vi "CPP_Aeroprobe_dT-Unified-kag.vi"() -> (5 "Plug in titles":string[](array[string]), 7 "Plug in values":string[](array[string]))   [LabVIEW 2016]
uses:
  ADAM Client/Sub VIs/ADAM Controls/Ch_description_ADAM.ctl
  ADAM Client/Sub VIs/ADAM Controls/Module_type_ADAM.ctl
  ADAM Client/Sub VIs/ADAM Controls/Function_ADAM.ctl
  ADAM Client/Sub VIs/ADAM Controls/Channel_State.ctl
  ADAM Client/Sub VIs/ADAM Controls/Calib_type_ADAM.ctl
  ADAM Client/Sub VIs/ADAM Controls/Address.ctl
  ADAM Client/Sub VIs/ADAM Controls/Update_scan_value.ctl
  <vilib>/Analysis/baseanly.llb/Mean (DBL).vi
  Globals/Constants_global.vi
  Globals/Meas_global.vi
  Globals/Trav_pos_global.vi
  <vilib>/Utility/file.llb/Write Delimited Spreadsheet (DBL).vi
  <vilib>/Analysis/NI_AALBase.lvlib
panel:
  out "MDZeroesVars":string[](array[string])
  out "MDZeroesMeans":string[](array[string])
  out "AeroFlow Output":cluster{string, string}[](array[cluster]) caption="Plug In Titles                                   Plug In Values"
  out "ZeroMeans&Vars":dbl[](array[numeric])
  out "ADAM Chs":T1[](array[typedef]) {"Duty" format="%.0b"; "D" format="%#_5g"; "C" format="%#_5g"; "B" format="%#_5g"; "A" format="%#_5g"}
  in  "Probe Orientation":u16(ring)=90 items=["Horizontal"=0, "Diagonal"=45, "Vertical"=90]
  in  "Probe Type":u16(ring)=12 items=["5-Hole Probe"=5, "OmniProbe"=12]
  in  "SaveTimeSeries?":bool
  in  "Mode":enum32{"Measure", "Take Zeroes"}(radio)
  in  "RunManually?":bool
  in  "MeanOrFull":bool
  in  "Graphs":bool
  in  "Downsampler":i32=80
  in  "Calibration Folder Path":path
  in  "Correction File Path":path
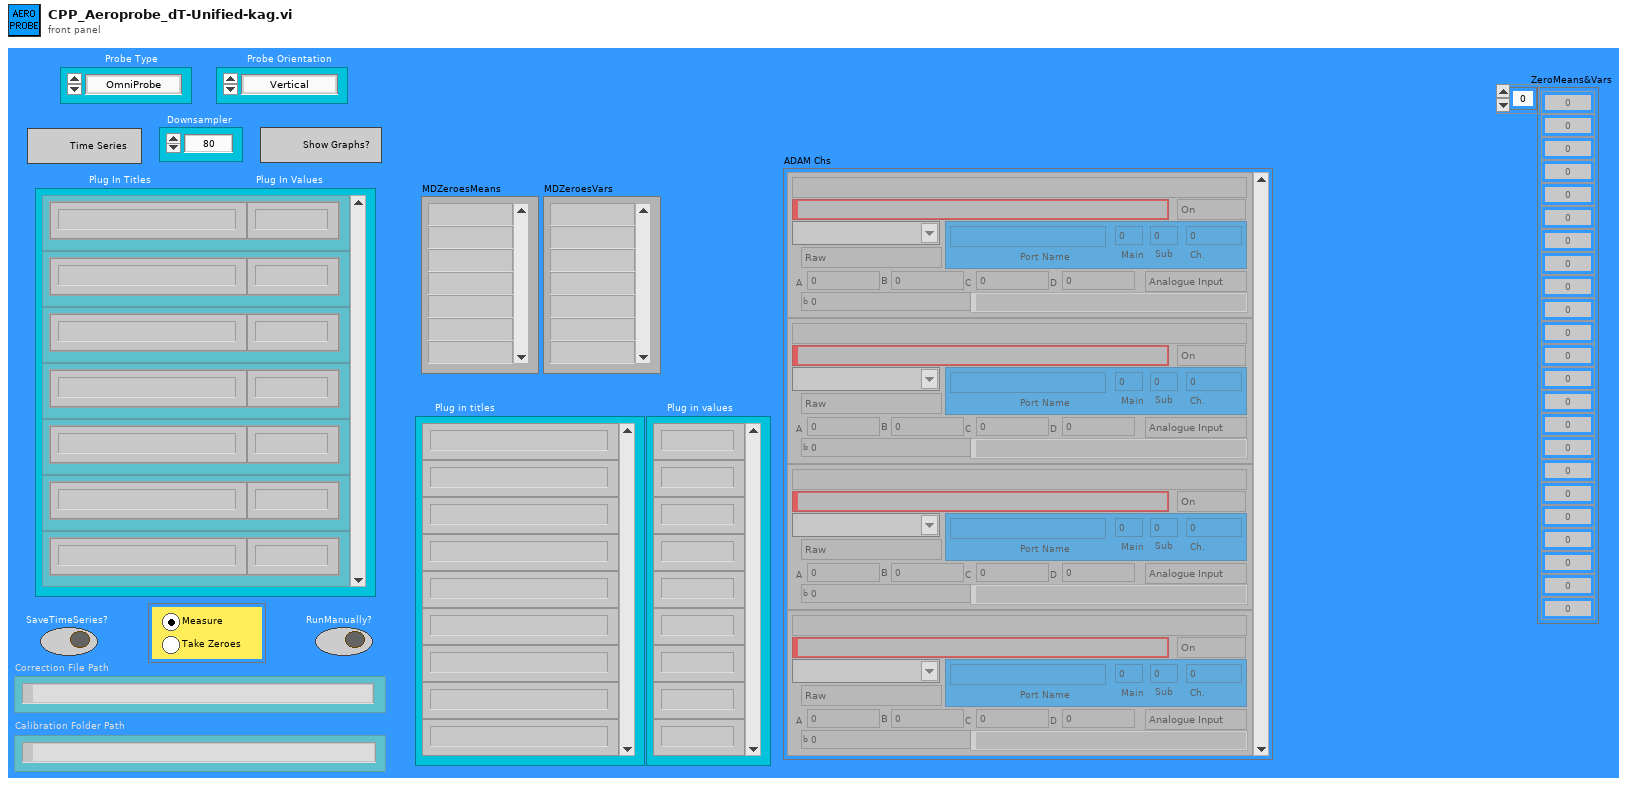
[diagram p1: front panel]
types:
  T1 = typedef "Ch_description_ADAM.ctl" = cluster{"Ch Name":string, "Type":T2, "Function":T3, "Ch State":T4, "Calibration type":T5, "A":dbl, "B":dbl, "C":dbl, "D":dbl, "Comments":string, "Address":T6, "String":string, "Duty":u16}
  T2 = typedef "Module_type_ADAM.ctl" = string
  T3 = typedef "Function_ADAM.ctl" = enum16{"Analogue Input", "Digital Input", "Event counter", "Event rate", "Analogue Output", "Digital Output", "Relay Output"}
  T4 = typedef "Channel_State.ctl" = enum16{"On", "Off", "Always On", "Always Off"}
  T5 = typedef "Calib_type_ADAM.ctl" = enum16{"Raw", "Bx + A", "Cx^2 + Bx + A", "Dx^3 + Cx^2 + Bx + A", "In Band", "Hi-Tec Q", "Hi-Tec M_dot", "Text"}
  T6 = typedef "Address.ctl" = cluster{"Main":i32, "Ch.":i32, "Sub":i32, "Port Name":string}
  T7 = enum16{"Save no data", "Save data in new files", "Save data in existing files"}
  T8 = typedef "Post_Process.ctl" = enum16{"Take New Data", "Post Process Raw Data File"}
  T9 = typedef "Analysis_info_cluster.ctl" = cluster{"Colour":u32, "Inst type":T10, "Inst name":string, "Symbol":string, "Code name":string, "Extra Info":string, "Inst Array":T11, "Extra Titles":string[], "Extra Values":string[], "U":dbl, "u^2":dbl, "u^3":dbl, "u^4":dbl, "Skew_u":dbl, "Kurt_u":dbl, "Sd Error in Mean":dbl, "% u'/U":dbl, "X":dbl, "Y":dbl, "Z":dbl, "Timescale integral to 25%":dbl, "Sd Error in Variance":dbl, "Calib File":path, "Calib Constants":dbl[], "Output Position":bool, "Full Stats":bool, "Av Sampling Rate":dbl, "Av No of Samples":dbl, "Total Meas Time (s)":dbl, "ADAM Ch Name":string, "Max value":dbl, "Min value":dbl}
  T10 = typedef "Inst_type.ctl" = enum16{"Propeller anemometer", "Raw voltage", "Pressure Transducer", "Pitot-static tube", "Preston tube", "Hot wire", "Cross wire 1", "Cross wire 2", "Generic Linear", "Generic Polynomial", "Generic BackPoly", "Fast FID", "Thermocouple", "Cold wire", "Pulsed Wire", "LDA Vel", "LDA Tran time", "LDA Arr time", "Microphone"}
  T11 = typedef "Instrument_Array.ctl" = enum16{"PWA", "LDA", "Analogue"}
  T12 = typedef "Traverse_cluster.ctl" = cluster{"Start X":sgl, "Start Y":sgl, "Start Z":sgl, "End X":sgl, "End Y":sgl, "End Z":sgl, "No. of pts.":i32, "Spacing":T13, "Filename":path, "Tunnel Speed":dbl, "Averaging time (min)":dbl, "Extra Commands":string, "Carrier_1 Q (l/min)":dbl, "Carrier_2 Q (l/min)":dbl, "Trace Gas Concentration (%)":dbl, "Specific Arguments":string, "Comments":string, "Row No":i32, "Row Type Selector":T14, "Completion time":string, "Row Duration (mins)":dbl, "No. of Valid pts.":i32, "Meas Setup File":string}
  T13 = typedef "Spacing.ctl" = enum16{"Linear", "Log", "Gauss", "Specified", "N/A"}
  T14 = typedef "Multi_run_mode.ctl" = enum16{"Move Traverse Only", "Set Tunnel Speed Only", "Set Source Only", "Set Measurement Conditions", "Single Measurement", "Vertical Profile", "Lateral Profile", "Longitudinal Profile", "Explore Volume", "Multi-Axis Profile", "Auto Calibrate", "Meas Fast FID Bkgnd", "Check Beam Power", "Scanning Valve Measurement", "Run VI Named:", "Set ADAM Ch", "Wait (minutes)", "Send Message", "Synchronize With:", "Fall Back to this Row", "Turn Off Row Repeating", "Blank Row", "Traverse 3D Volume"}
  T15 = typedef "Update_scan_value.ctl" = cluster{"Channel Name":string, "New Value":dbl}
  T16 = typedef "Time_Trace_Cluster.ctl" = cluster{"Weighting":dbl[], "Time (s)":dbl[], "Voltage":dbl[], "Eng Values":dbl[]}
  T17 = typedef "GoodArray.ctl" = bool[]
  T18 = typedef "SanityCluster.ctl" = cluster{"PressureErrors":bool[][], "Plug in titles":string[]}
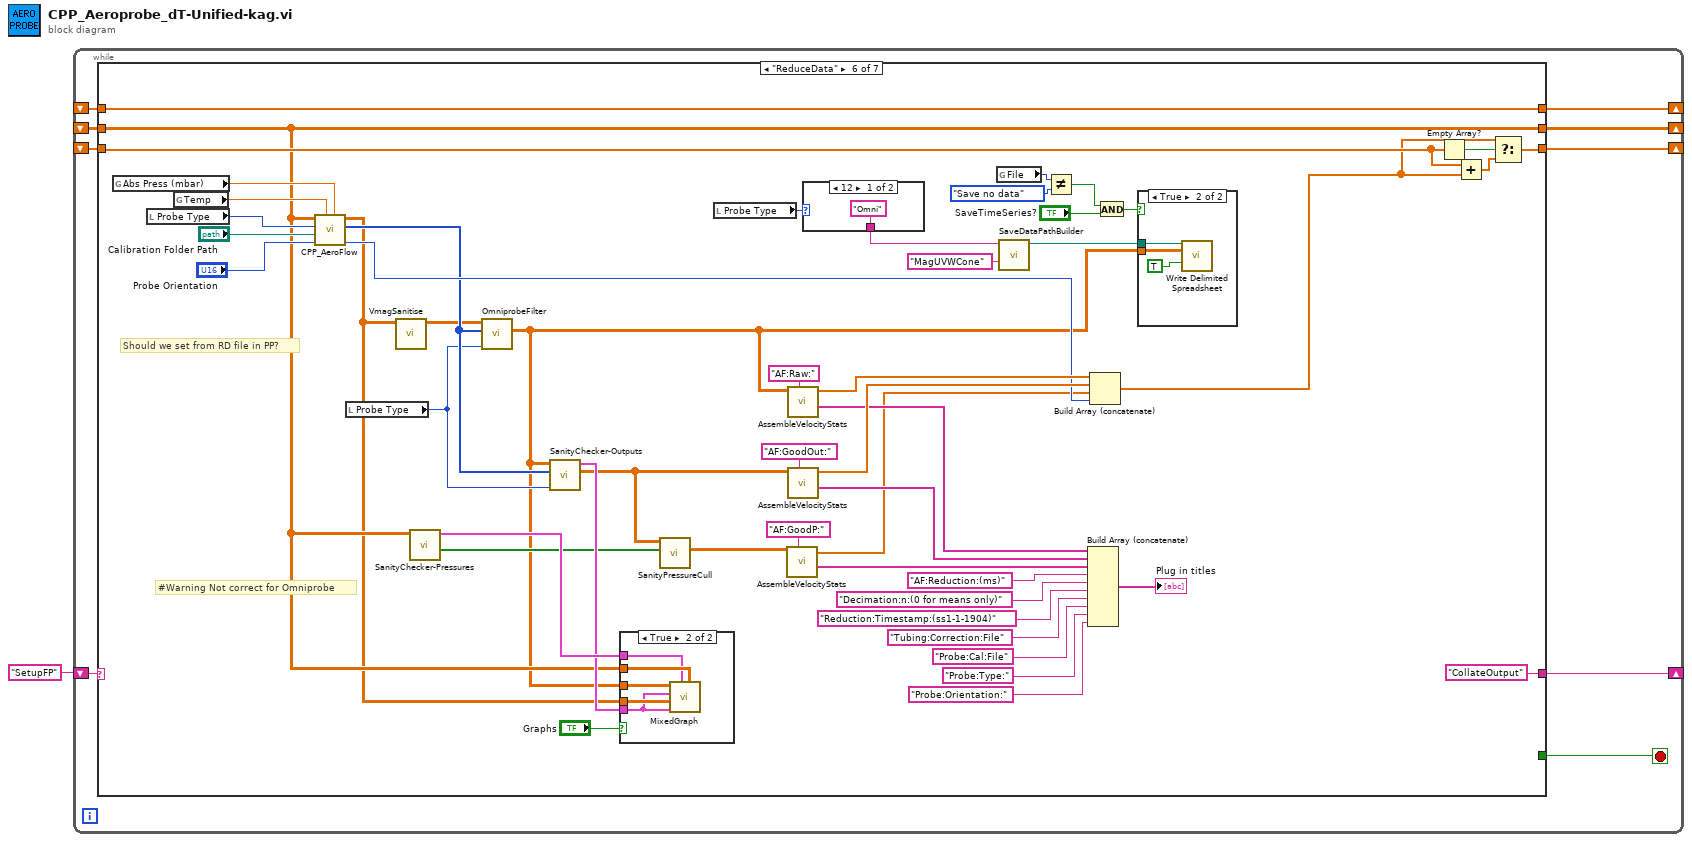
[diagram p0: block diagram]
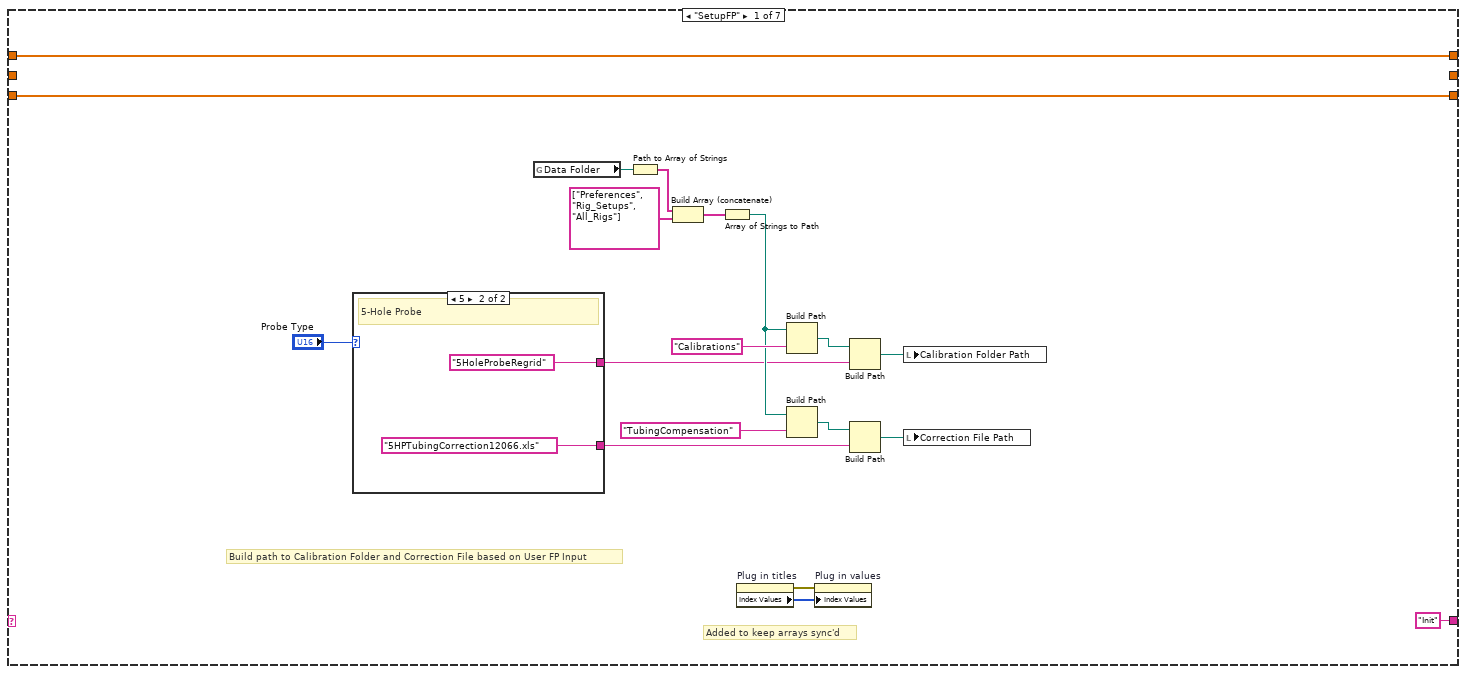
[diagram p2: hidden frame]
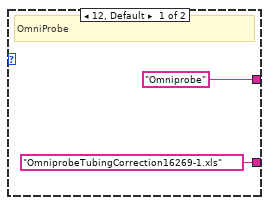
[diagram p3: hidden frame]
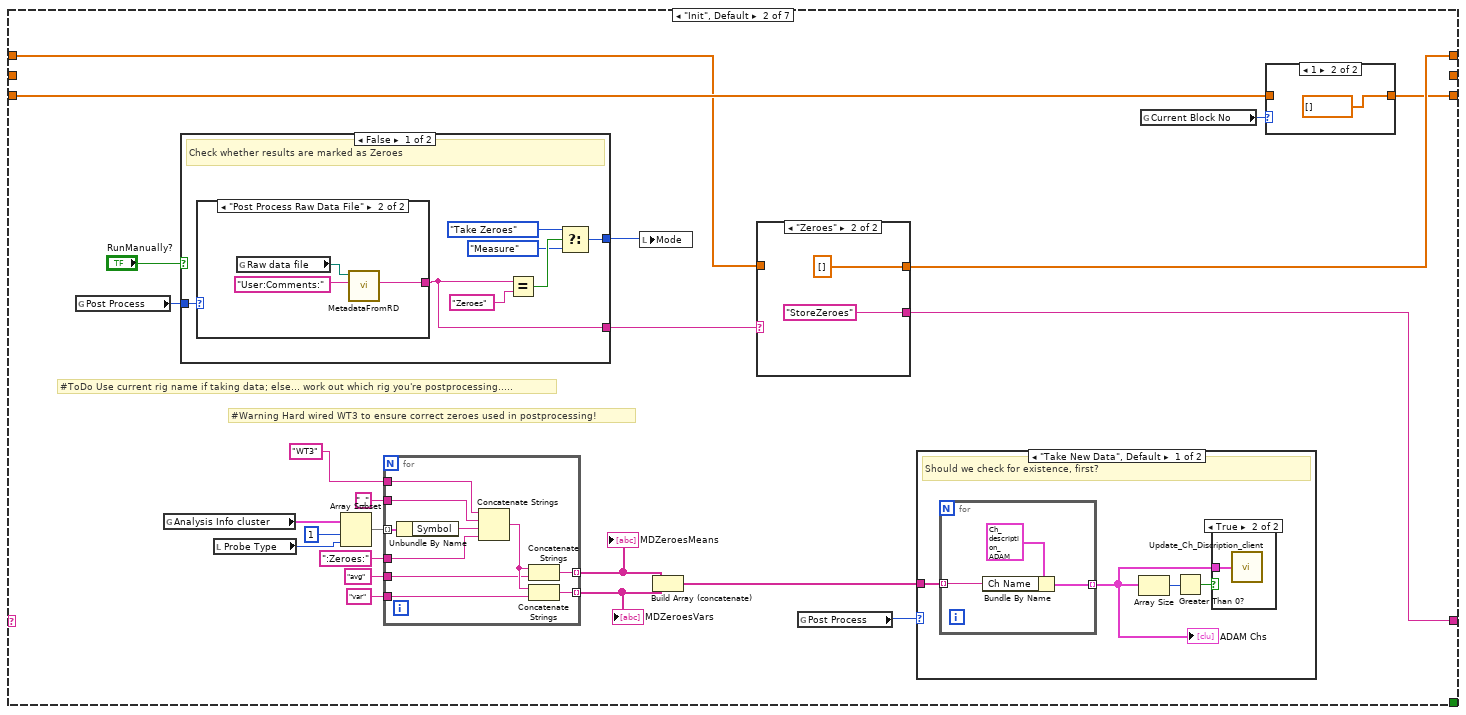
[diagram p4: hidden frame]
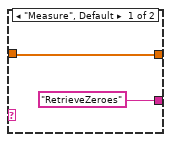
[diagram p7: hidden frame]
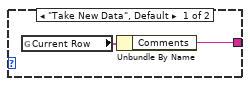
[diagram p8: hidden frame]
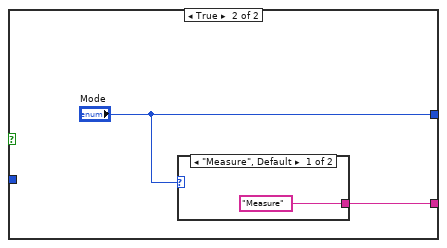
[diagram p9: hidden frame]
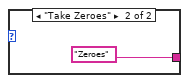
[diagram p10: hidden frame]
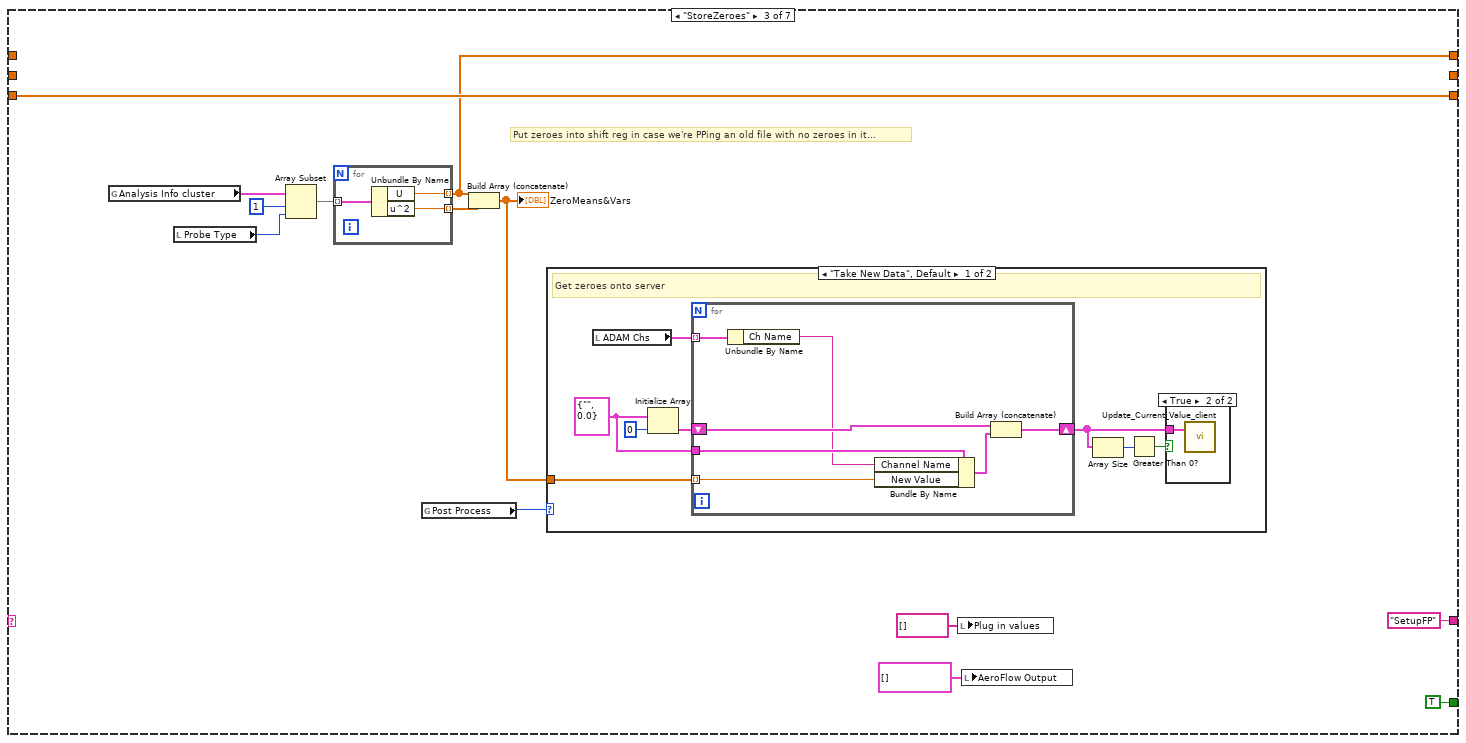
[diagram p12: hidden frame]
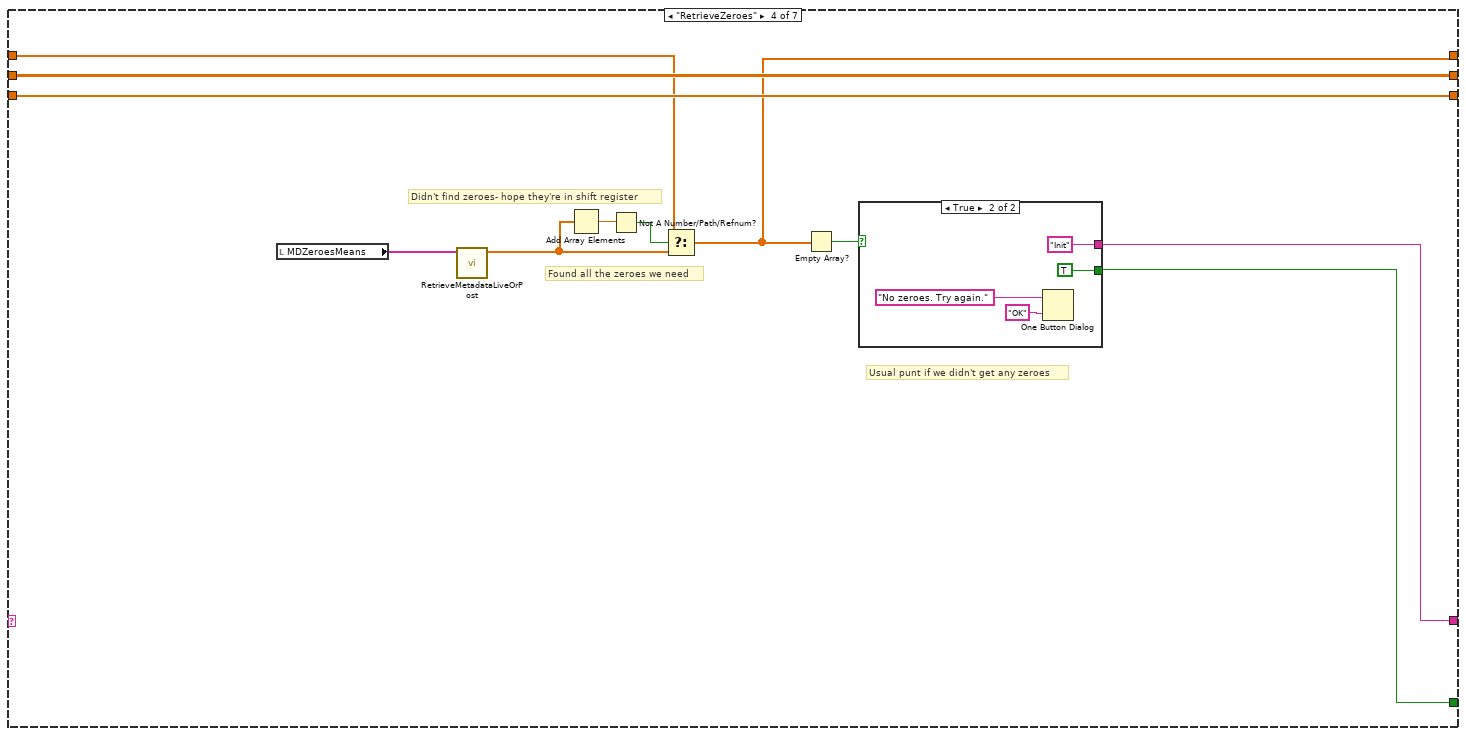
[diagram p15: hidden frame]
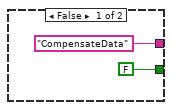
[diagram p16: hidden frame]
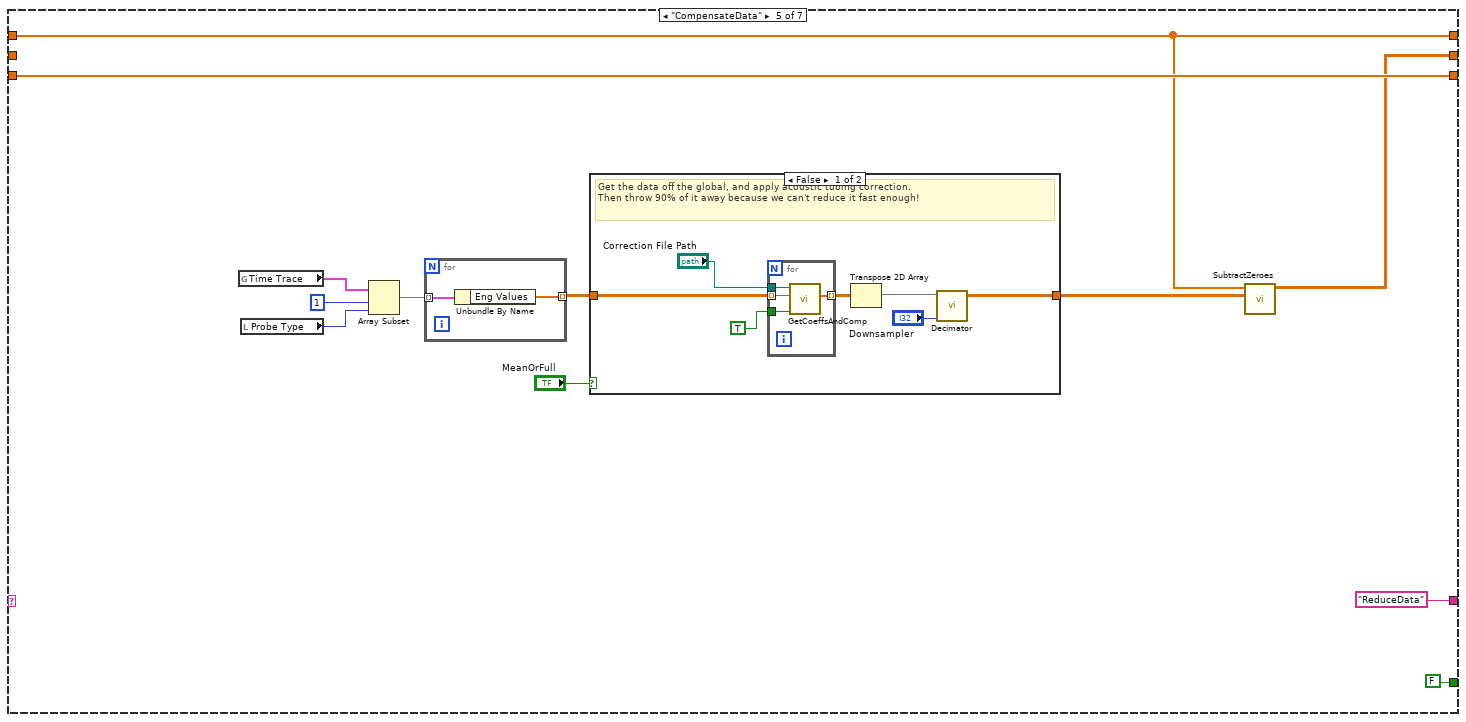
[diagram p17: hidden frame]
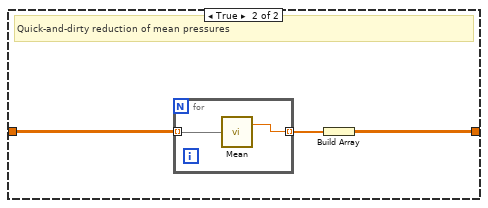
[diagram p18: hidden frame]
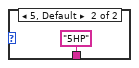
[diagram p19: hidden frame]
diagram:
  n1 = while {
    shift-right: [w9] -> _
    shift-left: "SetupFP" -> [w10]
    shift-right: [w8] -> _
    shift-left: _ -> [w7]
    shift-right: [w6] -> _
    shift-left: _ -> [w5]
    shift-right: [w3] -> _
    shift-left: _ -> [w2]
    stop <- w4 stop-if-true
    n2 = case shown="\"ReduceData\"" w10 {
      tunnel: ["Init" w39 "SetupFP" w134 "ReduceData" "CollateOutput" "Init"] -> w9
      tunnel: [w29 w56 w103 w129 w155 w225 w262] -> w8
      tunnel: w7 -> [w29 w40 _ w131 w155 w225 w262]
      tunnel: [w28 w55 w109 w139 w157 w221 w256] -> w6
      tunnel: w5 -> [w28 w54 w109 w139 w157 w224 w256]
      tunnel: [_ _ TRUE w133 FALSE _ TRUE] -> w4
      tunnel: [_ _ _ w138 w152 w181 w258] -> w3
      tunnel: w2 -> [_ _ _ w138 _ w181 w258]
      frame "SetupFP" {
        # "Added to keep arrays sync'd"
        # "Build path to Calibration Folder and Correction File based on User FP Input"
        n3 = case shown="5" "Probe Type" {
          tunnel: ["OmniprobeTubingCorrection16269-1.xls" ("Tubing Compensation File") "5HPTubingCorrection12066.xls" ("Tubing Compensation File")] -> w18
          tunnel: ["Omniprobe" ("Calibration Folder") "5HoleProbeRegrid" ("Calibration Folder")] -> w17
          frame 12, Default {
            # "OmniProbe"
          }
          frame 5 {
            # "5-Hole Probe"
          }
        }
        n4 = global read "Constants_global.vi" "Data Folder"() -> (w23:path)
        n5 = Path to Array of Strings(0:w23) -> (2:w26:string[])  [unwired: 1 out]
        n6 = Build Array (concatenate)(w26, string[] ["Preferences", "Rig_Setups", "All_Rigs"] ("array of strings 3")) -> (w24:string[])
        n7 = Array of Strings to Path(0:w24) -> (2:w20:path)  [unwired: 1 in]
        n8 = property on="Plug in titles" class="Arr (strict)"() -> (error out=w11:errorcluster, "Index Values"=w12:u32[])  [unwired: 2 in, 1 out]
        n9 = Build Path(base path=w20, name or relative path="Calibrations") -> (appended path=w15:path)
        n10 = Build Path(base path=w20, name or relative path="TubingCompensation") -> (appended path=w16:path)
        n11 = property on="Plug in values" class="Arr (strict)"(error in=w11, "Index Values"=w12) -> ()  [unwired: 1 in, 2 out]
        n12 = Build Path(base path=w15, name or relative path=w17) -> (appended path=w14:path)
        n13 = Build Path(base path=w16, name or relative path=w18) -> (appended path=w13:path)
        n14 = local write "Calibration Folder Path"(w14) -> ()
        n15 = local write "Correction File Path"(w13) -> ()
      }
      frame "Init", Default {
        # "#ToDo Use current rig name if taking data; else... work out which rig you're postprocessing....."
        # "#Warning Hard wired WT3 to ensure correct zeroes used in postprocessing!"
        n16 = global read "Meas_global.vi" "Post Process"() -> (w50:T8)
        n17 = global read "Meas_global.vi" "Analysis Info cluster"() -> (w48:T9[])
        n18 = case shown="False" "RunManually?" {
          tunnel: [w85 "Mode"] -> w51
          tunnel: w50 -> [w80 _]
          tunnel: [w79 w91] -> w41
          frame False {
            # "Check whether results are marked as Zeroes"
            n19 = case shown="\"Post Process Raw Data File\"" w80 {
              tunnel: [w86 w88] -> w79
              frame "Take New Data", Default {
                n20 = global read "Trav_pos_global.vi" "Current Row"() -> (w87:T12)
                n21 = Unbundle By Name(w87) -> ("Comments"=w86:string)
              }
              frame "Post Process Raw Data File" {
                n22 = global read "Meas_global.vi" "Raw data file"() -> (w90:path)
                n23 = call "MetadataFromRD.vi"("ChannelName"="User:Comments:", "Raw data file"=w90) -> ("ValueString"=w88:string)  [unwired: 8 in, 1 out]
              }
            }
            n24 = Equal?(x=w79, y="Zeroes") -> (x = y?=w83:bool)
            n25 = Select(t=enum32{"Measure", "Take Zeroes"}."Take Zeroes" ("Mode"), s=w83, f=enum32{"Measure", "Take Zeroes"}."Measure" ("Mode")) -> (s? t:f=w85:enum32{"Measure", "Take Zeroes"})
          }
          frame True {
            n26 = case shown="\"Measure\", Default" "Mode" {
              tunnel: ["Measure" ("y") "Zeroes" ("y")] -> w91
              frame "Measure", Default {
              }
              frame "Take Zeroes" {
              }
            }
          }
        }
        n27 = local read "Probe Type"() -> (w42:u16)
        n28 = Array Subset(array=w48, index=1, length=w42) -> (w47:T9[])
        n29 = for {
          tunnel: w47 -> [w78] mode=indexing
          tunnel: ":Zeroes:" -> [w76]
          tunnel: "avg" -> [w73]
          tunnel: "var" -> [w75]
          tunnel: "_" -> [w72]
          tunnel: "WT3" -> [w71]
          tunnel: [w70] -> w37 mode=indexing
          tunnel: [w69] -> w36 mode=indexing
          n30 = Unbundle By Name(w78) -> ("Symbol"=w77:string)
          n31 = Concatenate Strings(w71, w72, w77, w76) -> (w74:string)
          n32 = Concatenate Strings(w74, w73) -> (w70:string)
          n33 = Concatenate Strings(w74, w75) -> (w69:string)
        }
        "MDZeroesMeans" <- w37
        "MDZeroesVars" <- w36
        n34 = local write "Mode"(w51) -> ()
        n35 = Build Array (concatenate)(w37, w36) -> (w35:string[])
        n36 = case shown="\"Zeroes\"" w41 {
          tunnel: [w66 dbl[] [] ("t")] -> w56
          tunnel: w40 -> [w66 _]
          tunnel: ["RetrieveZeroes" "StoreZeroes"] -> w39
          frame "Measure", Default {
          }
          frame "Zeroes" {
          }
        }
        n37 = global read "Meas_global.vi" "Post Process"() -> (w38:T8)
        n38 = case shown="\"Take New Data\", Default" w38 {
          tunnel: w35 -> [w60 _]
          frame "Take New Data", Default {
            # "Should we check for existence, first?"
            n39 = for {
              tunnel: w60 -> [w63] mode=indexing
              tunnel: [w62] -> w57 mode=indexing
              n40 = Bundle By Name(cluster=T1 {"Ch Name"="", "Type"="Hold Value", "Function"=enum."Analogue Input", "Ch State"=enum."On", "Calibration type"=enum."Raw", "A"=0.0, "B"=0.0, "C"=0.0, "D"=0.0, "Comments"="", "Address"={"Main"=0, "Ch."=0, "Sub"=0, "Port Name"=""}, "String"="", "Duty"=0} ("Ch Discription"), "Ch Name"=w63) -> (w62:T1)
            }
            "ADAM Chs" <- w57
            n41 = Array Size(array=w57) -> (size(s)=w59:i32)
            n42 = Greater Than 0?(x=w59) -> (x > 0?=w58:bool)
            n43 = case shown="True" w58 {
              tunnel: w57 -> [_ w61]
              frame False {
              }
              frame True {
                n44 = call "Update_Ch_Discription_client.vi"("Channels to update In"=w61) -> ()  [unwired: 1 out]
              }
            }
          }
          frame "Post Process Raw Data File" {
          }
        }
        n45 = global read "Meas_global.vi" "Current Block No"() -> (w53:i32)
        n46 = case shown="1" w53 {
          tunnel: [w95 dbl[] [] ("t")] -> w55
          tunnel: w54 -> [w95 _]
          frame 0, Default {
          }
          frame 1 {
          }
        }
      }
      frame "StoreZeroes" {
        # "Put zeroes into shift reg in case we're PPing an old file with no zeroes in it..."
        n47 = global read "Meas_global.vi" "Analysis Info cluster"() -> (w107:T9[])
        n48 = local read "Probe Type"() -> (w105:u16)
        n49 = Array Subset(array=w107, index=1, length=w105) -> (w106:T9[])
        n50 = for {
          tunnel: w106 -> [w128] mode=indexing
          tunnel: [w127] -> w103 mode=indexing
          tunnel: [w126] -> w104 mode=indexing
          n51 = Unbundle By Name(w128) -> ("U"=w127:dbl, "u^2"=w126:dbl)
        }
        n52 = global read "Meas_global.vi" "Post Process"() -> (w101:T8)
        n53 = Build Array (concatenate)(w103, w104) -> (w102:dbl[])
        "ZeroMeans&Vars" <- w102
        n54 = case shown="\"Take New Data\", Default" w101 {
          tunnel: w102 -> [w110 _]
          frame "Take New Data", Default {
            w112 = T15 {"Channel Name"="", "New Value"=0.0} ("Update Scan Value Cluster")
            # "Get zeroes onto server"
            n55 = local read "ADAM Chs"() -> (w111:T1[])
            n56 = Initialize Array(w112, 0 ("Dimension Size")) -> (w116:T15[])
            n57 = for {
              shift-right: [w125] -> w113
              shift-left: w116 -> [w124]
              tunnel: w110 -> [w122] mode=indexing
              tunnel: w111 -> [w121] mode=indexing
              tunnel: w112 -> [w123]
              n58 = Unbundle By Name(w121) -> ("Ch Name"=w120:string)
              n59 = Bundle By Name(cluster=w123, "Channel Name"=w120, "New Value"=w122) -> (w119:T15)
              n60 = Build Array (concatenate)(w124, w119) -> (w125:T15[])
            }
            n61 = Array Size(array=w113) -> (size(s)=w114:i32)
            n62 = Greater Than 0?(x=w114) -> (x > 0?=w115:bool)
            n63 = case shown="True" w115 {
              tunnel: w113 -> [_ w118]
              frame False {
              }
              frame True {
                n64 = call "Update_Current_Value_client.vi"("Update array in"=w118) -> ()  [unwired: 1 in]
              }
            }
          }
          frame "Post Process Raw Data File" {
            # "-or, if they're not in the file, it's old data, and we'll use the ones we stuck in the shift register up there^...."
            # "Zeroes will already be in file"
          }
        }
        n65 = local write "Plug in values"(string[] [] ("Plug in values")) -> ()
        n66 = local write "AeroFlow Output"(cluster{string, string}[] [] ("AeroFlow Output")) -> ()
      }
      frame "RetrieveZeroes" {
        # "Didn't find zeroes- hope they're in shift register"
        # "Found all the zeroes we need"
        # "Usual punt if we didn't get any zeroes"
        n67 = local read "MDZeroesMeans"() -> (w137:string[])
        n68 = call "RetrieveMetadataLiveOrPost.vi"("ChannelsToGet"=w137) -> ("ChannelValues"=w130:dbl[])  [unwired: 10 in]
        n69 = Add Array Elements(numeric array=w130) -> (sum=w136:dbl)
        n70 = Not A Number/Path/Refnum?(number/path/refnum=w136) -> (NaN/Path/Refnum?=w132:bool)
        n71 = Select(t=w131, s=w132, f=w130) -> (s? t:f=w129:dbl[])
        n72 = Empty Array?(array=w129) -> (empty?=w135:bool)
        n73 = case shown="True" w135 {
          tunnel: ["CompensateData" "Init"] -> w134
          tunnel: [FALSE TRUE] -> w133
          frame False {
          }
          frame True {
            n74 = One Button Dialog(message="No zeroes. Try again.", button name ("OK")="OK") -> ()  [unwired: 1 out]
          }
        }
      }
      frame "CompensateData" {
        n75 = global read "Meas_global.vi" "Time Trace"() -> (w150:T16[])
        n76 = local read "Probe Type"() -> (w146:u16)
        n77 = Array Subset(array=w150, index=1, length=w146) -> (w148:T16[])
        n78 = for {
          tunnel: w148 -> [w159] mode=indexing
          tunnel: [w158] -> w147 mode=indexing
          n79 = Unbundle By Name(w159) -> ("Eng Values"=w158:dbl[])
        }
        n80 = case shown="False" "MeanOrFull" {
          tunnel: [w161 w173] -> w156
          tunnel: w147 -> [w160 w172]
          frame False {
            # "Get the data off the global, and apply acoustic tubing correction. \nThen throw 90% of it away because we can't reduce it fast enough!"
            n81 = for {
              tunnel: w160 -> [w170] mode=indexing
              tunnel: [w169] -> w164 mode=indexing
              tunnel: TRUE ("Apply Phase Correction?") -> [w168]
              tunnel: "Correction File Path" -> [w167]
              n82 = call "GetCoeffsAndComp.vi"("Apply Phase Correction?"=w168, "mutedData"=w170, "TubingCorrectionFile"=w167) -> ("boostedData"=w169:dbl[])  [unwired: 8 in]
            }
            n83 = Transpose 2D Array(2D array=w164) -> (transposed array=w163:dbl[][])
            n84 = call "Decimator.vi"("Decimator"="Downsampler", "Array In"=w163) -> ("DecimatedArrayOut"=w161:dbl[][])  [unwired: 9 in]
          }
          frame True {
            # "Quick-and-dirty reduction of mean pressures"
            n85 = for {
              tunnel: w172 -> [w175] mode=indexing
              tunnel: [w174] -> w171 mode=indexing
              n86 = call-poly <vilib>:"Mean.vi"("X"=w175) -> ("mean"=w174:dbl)  [unwired: 1 out]
            }
            n87 = Build Array(w171) -> (w173:dbl[][])
          }
        }
        n88 = call "SubtractZeroes.vi"("RawPressure"=w156, "Zeroes"=w155) -> ("ZeroedPressure"=w152:dbl[][])  [unwired: 9 in]
      }
      frame "ReduceData" {
        # "Should we set from RD file in PP?"
        # "#Warning Not correct for Omniprobe"
        n89 = global read "Meas_global.vi" "Abs Press (mbar)"() -> (w219:dbl)
        n90 = local read "Probe Type"() -> (w184:u16)
        n91 = global read "Meas_global.vi" "Temp"() -> (w218:dbl)
        n92 = call "CPP_AeroFlow.vi"("Pressure (mBar)"=w219, "Temperature (C)"=w218, "Probe Orientation"="Probe Orientation", "Calibration Folder Path"="Calibration Folder Path", "Probe Type"=w184, "ZeroedPressures (mmH2O)"=w181) -> ("Time(ms)"=w207:u32, "ReductionCode"=w180:i32[], "RawVmagUVWCone"=w176:dbl[][])  [unwired: 1 out]
        n93 = local read "Probe Type"() -> (w179:u16)
        n94 = call "VmagSanitise.vi"("RawVmagUVWCone"=w176) -> ("NaNsanitisedVmagUVWCone"=w178:dbl[][])  [unwired: 10 in]
        n95 = call "SanityChecker-Pressures.vi"("ZeroedPressures"=w181) -> ("GoodPressures"=w203:T17, "Sanity"=w215:T18)  [unwired: 9 in]
        n96 = call "OmniprobeFilter.vi"("Probe Type"=w179, "ReductionCode"=w180, "RawVmagUVWCone"=w178) -> ("FilteredVmagUVWCone"=w177:dbl[][])  [unwired: 8 in]
        n97 = call "SanityChecker-Outputs.vi"("Probe Type"=w179, "ReductionCode"=w180, "RawVmagUVWCone"=w177) -> ("SanitisedVmagUVWCone"=w204:dbl[][], "OutputErrors"=w214:T18)  [unwired: 5 in, 2 out]
        n98 = case shown="True" "Graphs" {
          tunnel: w181 -> [_ w236]
          tunnel: w215 -> [_ w235]
          tunnel: w176 -> [_ w234]
          tunnel: w214 -> [_ w232]
          tunnel: w177 -> [_ w233]
          frame False {
          }
          frame True {
            n99 = call "MixedGraph.vi"("ZeroedPressure"=w236, "PressureSanity"=w235, "OutputErrors2"=w232, "RawVmagUVWCone2"=w234, "OutputErrors1"=w232, "RawVmagUVWCone1"=w233) -> ()  [unwired: 6 in]
          }
        }
        n100 = call "SanityPressureCull.vi"("GoodPressures"=w203, "VmagUVWCone"=w204) -> ("SanitisedVmagUVWCone"=w205:dbl[][])  [unwired: 9 in]
        n101 = local read "Probe Type"() -> (w183:u16)
        n102 = call "AssembleVelocityStats.vi"("TitlePrefix"="AF:GoodP:", "VmagUVWCone"=w205) -> ("Plug in titles"=w202:string[], "StatsArray"=w200:dbl[])  [unwired: 8 in]
        n103 = call "AssembleVelocityStats.vi"("TitlePrefix"="AF:Raw:", "VmagUVWCone"=w177) -> ("Plug in titles"=w209:string[], "StatsArray"=w211:dbl[])  [unwired: 8 in]
        n104 = call "AssembleVelocityStats.vi"("TitlePrefix"="AF:GoodOut:", "VmagUVWCone"=w204) -> ("Plug in titles"=w208:string[], "StatsArray"=w210:dbl[])  [unwired: 8 in]
        n105 = case shown="12" w183 {
          tunnel: ["Omni" ("Inst name") "5HP" ("Inst name")] -> w182
          frame 12 {
          }
          frame 5, Default {
          }
        }
        n106 = global read "Meas_global.vi" "File"() -> (w192:T7)
        n107 = call "SaveDataPathBuilder.vi"("DataTypeSuffix"="MagUVWCone", "Inst name"=w182) -> ("Path name Out"=w194:path)  [unwired: 9 in]
        n108 = Not Equal?(x=w192, y=T7."Save no data" ("File")) -> (x != y?=w189:bool)
        n109 = Build Array (concatenate)(w209, w208, w202, "AF:Reduction:(ms)", "Decimation:n:(0 for means only)" ("element"), "Reduction:Timestamp:(ss1-1-1904)" ("element"), "Tubing:Correction:File" ("element"), "Probe:Cal:File" ("element"), "Probe:Type:" ("element"), "Probe:Orientation:" ("element")) -> (→"Plug in titles":string[])
        n110 = Build Array (concatenate)(w211, w210, w200, w207) -> (w212:dbl[])
        n111 = And(x=w189, y="SaveTimeSeries?") -> (x .and. y?=w190:bool)
        n112 = case shown="True" w190 {
          tunnel: w177 -> [_ w230]
          tunnel: w194 -> [_ w231]
          frame False {
          }
          frame True {
            n113 = call-poly <vilib>:"Write Delimited Spreadsheet.vi"("file path (dialog if empty)"=w231, "2D data"=w230, "append to file? (new file:F)"=TRUE) -> ()  [unwired: 11 in, 2 out]
          }
        }
        n114 = Empty Array?(array=w224) -> (empty?=w223:bool)
        n115 = Add(x=w224, y=w212) -> (x+y=w222:dbl[])
        n116 = Select(t=w212, s=w223, f=w222) -> (s? t:f=w221:dbl[])
      }
      frame "CollateOutput" {
        # "Calculate ensemble average"
        n117 = global read "Meas_global.vi" "Current Block No"() -> (w259:i32)
        n118 = local read "Downsampler"() -> (w255:i32)
        n119 = local read "MeanOrFull"() -> (w254:bool)
        n120 = local read "Calibration Folder Path"() -> (w244:path)
        n121 = local read "Correction File Path"() -> (w246:path)
        n122 = Divide(x=w256, y=w259) -> (x/y=w257:dbl[])
        n123 = Get Date/Time In Seconds() -> (seconds since 1Jan1904=w251:timestamp)
        n124 = Number To Decimal String(number=w255) -> (decimal integer string=w253:string)  [unwired: 1 in]
        n125 = property on="Probe Type" class="Ring (strict)"() -> ("RingText.Text"=w241:string)  [unwired: 2 in, 2 out]
        n126 = property on="Probe Orientation" class="Ring (strict)"() -> ("RingText.Text"=w240:string)  [unwired: 2 in, 2 out]
        n127 = To Double Precision Float(number=w251) -> (double precision float=w250:dbl)
        n128 = Number To Fractional String(number=w257) -> (F-format string=w247:string[])  [unwired: 3 in]
        n129 = Select(t="0", s=w254, f=w253) -> (s? t:f=w249:string)
        n130 = Number To Fractional String(number=w250, precision (6)=i16 3) -> (F-format string=w248:string)  [unwired: 2 in]
        n131 = Path To String(path=w246) -> (string=w245:string)
        n132 = Path To String(path=w244) -> (string=w243:string)
        n133 = Build Array (concatenate)(w247, w249, w248, w245, w243, w241, w240) -> (w239:string[])
        "Plug in values" <- w239
        n134 = local read "Plug in titles"() -> (w238:string[])
        n135 = for {
          tunnel: w239 -> [w265] mode=indexing
          tunnel: w238 -> [w264] mode=indexing
          tunnel: [w263] -> w237 mode=indexing
          n136 = Bundle(w264, "RingText.Text"=w265) -> (w263:cluster{string, "RingText.Text":string})  [unwired: 1 in]
        }
        "AeroFlow Output" <- w237
      }
    }
  }
